vi "Whole map lib.vi"(6 "stop":bool, 8 "error in (no error)":errorcluster, 9 "sensor y":fxp<+/-,64,32>, 10 "Sensor x":fxp<+/-,64,32>, 11 "map reference in":refnum<data-value>) -> (0 "error out":errorcluster, 3 "map reference out 2":refnum<data-value>)   [LabVIEW 2012]
uses:
  <vilib>/robotics/Navigation/shared/WorldMap/OccupancyGridWorldMap/NI_Robotics_OccupancyGridWorldMap.lvclass
  <vilib>/rvi/interface/nirviOpenFPGA/nirviOpenFPGA.xnode
  <vilib>/rvi/interface/nirviReadWriteControl/nirviReadWriteControl.xnode
  <vilib>/rvi/interface/nirviCloseFPGA/nirviCloseFPGA.xnode
  <vilib>/FPGAPlugInAG/Dynamic/niLvFpga_Close_Dynamic.vi
  NiFpgaLv.dll
  <vilib>/Utility/error.llb/Error Cluster From Error Code.vi
  <vilib>/rvi/interface/Simulation/niFpgaSimulationCallBeginRW.vi
  <vilib>/rvi/errors/niLvFpgaAdjustHostInterfaceError.vi
  fpgatrig.vi
  <vilib>/rvi/interface/RandomDataEmulation/nirviRandomDataOpen.vi
  <vilib>/rvi/interface/common/niFpgaCacheSessionInfoDynamic.vi
panel:
  in  "distance":fxp<+/-,64,32>
  in  "Degrees":dbl
  out "Rounded y":fxp<+/-,64,32>
  out "Rounded x":fxp<+/-,64,32>
  out "Detected x":fxp<+/-,64,32>
  out "Detected y":fxp<+/-,64,32>
  # "Add into own loop so it updates map independent of disicion making"
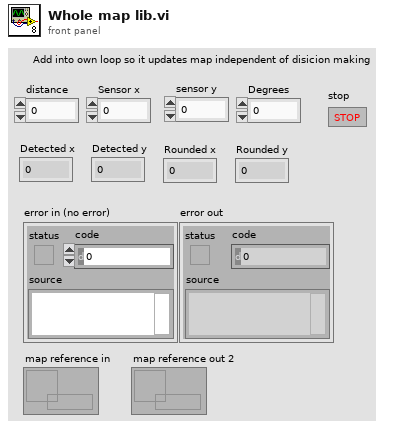
[diagram p1: front panel]
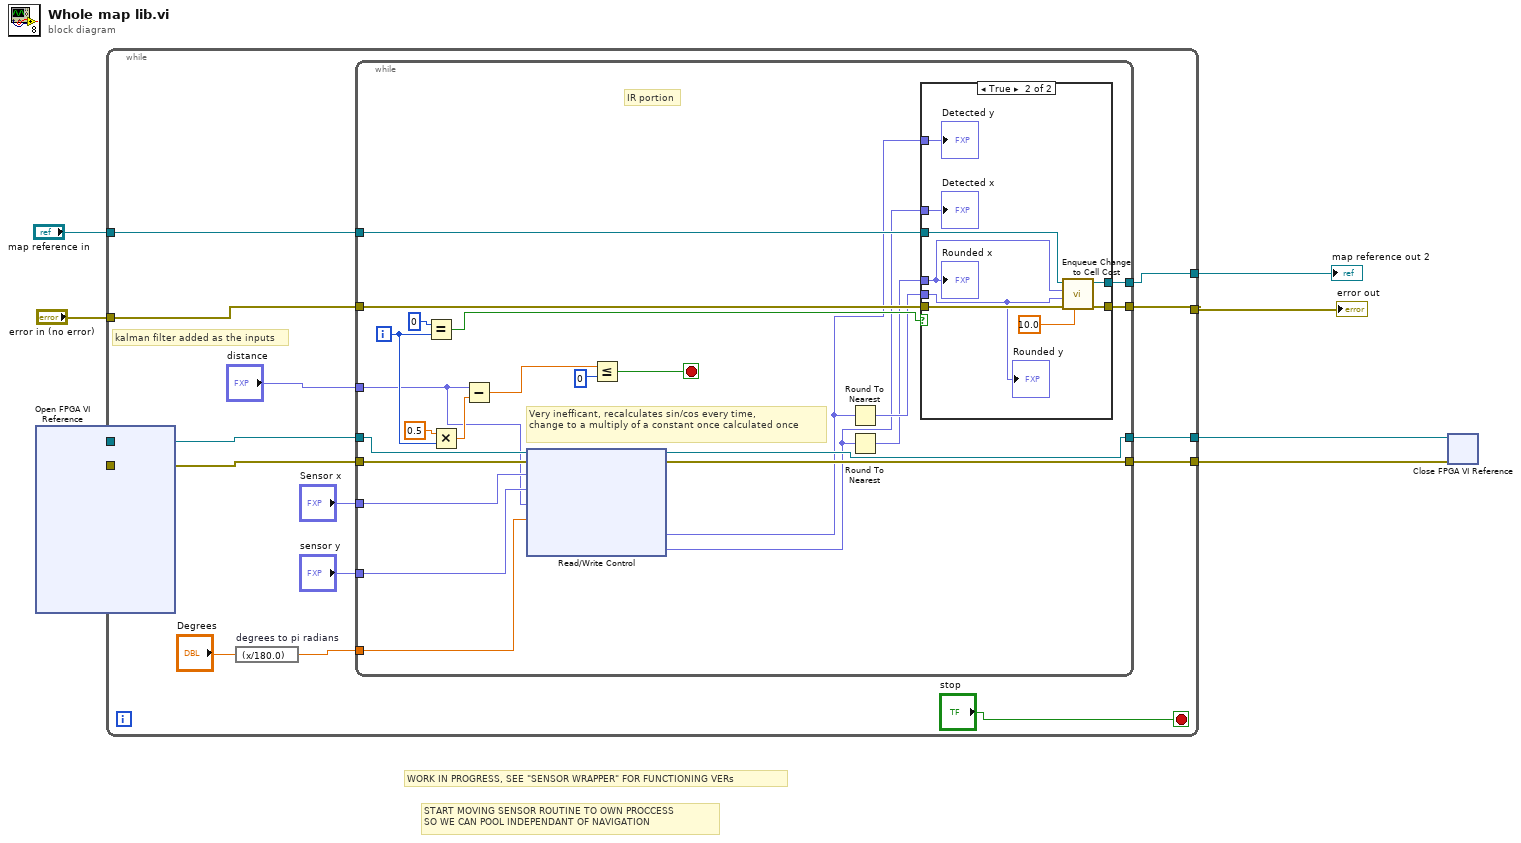
[diagram p0: block diagram]
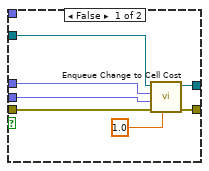
[diagram p2: hidden frame]
diagram:
  # "WORK IN PROGRESS, SEE \"SENSOR WRAPPER\" FOR FUNCTIONING VERs"
  # "START MOVING SENSOR ROUTINE TO OWN PROCCESS\nSO WE CAN POOL INDEPENDANT OF NAVIGATION"
  n1 = xnode "Open FPGA VI Reference"() -> ("FPGA VI Reference Out"=w3:refnum<k20>, "error out"=w4:errorcluster)  [unwired: 2 in]
  n2 = while {
    tunnel: [w19] -> w8
    tunnel: [w18] -> w7
    tunnel: "map reference in" -> [w17]
    tunnel: "error in (no error)" -> [w16]
    tunnel: w4 -> [w13]
    tunnel: w3 -> [w12]
    tunnel: [w11] -> w2
    tunnel: [w10] -> w1
    stop <- "stop" stop-if-true
    # "kalman filter added as the inputs"
    n3 = expression code="(x/180.0)" "degrees to pi radians"("Degrees") -> (w14:dbl)
    n4 = while {
      tunnel: w17 -> [w46]
      tunnel: w16 -> [w45]
      tunnel: [w44] -> w19
      tunnel: [w43] -> w18
      tunnel: "sensor y" -> [w25]
      tunnel: "Sensor x" -> [w24]
      tunnel: w14 -> [w27]
      tunnel: "distance" -> [w23]
      tunnel: w13 -> [w33]
      tunnel: w12 -> [w32]
      tunnel: [w31] -> w11
      tunnel: [w30] -> w10
      i -> [w38]
      stop <- w34 stop-if-true
      # "IR portion"
      # "Very inefficant, recalculates sin/cos every time, \nchange to a multiply of a constant once calculated once"
      n5 = Equal?(x=0, y=w38) -> (x = y?=w41:bool)
      n6 = Multiply(x=0.5, y=w38) -> (x*y=w36:dbl)
      n7 = Subtract(x=w23, y=w36) -> (x-y=w26:dbl)
      n8 = xnode "Read/Write Control"("FPGA VI Reference In"=w32, "error in"=w33, "Sensor position x"=w24, "Sensor position y"=w25, "Distance detected"=w23, "sensor angle (Radiens)"=w27) -> ("FPGA VI Reference Out"=w31:refnum<k20>, "error out"=w30:errorcluster, "Detected y Cord"=w29:fxp<+/-,64,32>, "Detected x Cord"=w28:fxp<+/-,64,32>)
      n9 = Less Or Equal?(x=w26, y=0) -> (x <= y?=w34:bool)
      n10 = Round To Nearest(number=w29) -> (nearest integer value=w40:fxp<+/-,33,33>)
      n11 = Round To Nearest(number=w28) -> (nearest integer value=w39:fxp<+/-,33,33>)
      n12 = case shown="True" w41 {
        tunnel: w46 -> [w49 w62]
        tunnel: w45 -> [w50 w61]
        tunnel: [w52 w59] -> w44
        tunnel: [w51 w58] -> w43
        tunnel: w39 -> [w48 w54]
        tunnel: w40 -> [w47 w55]
        tunnel: w28 -> [_ w57]
        tunnel: w29 -> [_ w56]
        frame False {
          n13 = call <vilib>:"Enqueue Change to Cell Cost.vi"("cost"=1.0, "error in (no error)"=w50, "y"=w47, "x"=w48, "map reference in"=w49) -> ("error out"=w51:errorcluster, "map reference out"=w52:refnum<data-value>)  [unwired: 5 in]
        }
        frame True {
          n14 = call <vilib>:"Enqueue Change to Cell Cost.vi"("cost"=10.0, "error in (no error)"=w61, "y"=w55, "x"=w54, "map reference in"=w62) -> ("error out"=w58:errorcluster, "map reference out"=w59:refnum<data-value>)  [unwired: 5 in]
          "Rounded y" <- w55
          "Rounded x" <- w54
          "Detected x" <- w57
          "Detected y" <- w56
        }
      }
    }
  }
  "map reference out 2" <- w8
  "error out" <- w7
  n15 = xnode "Close FPGA VI Reference"("FPGA VI Reference In"=w2, "error in"=w1) -> ()  [unwired: 1 out]
